vi "Imaging Data Display.vi"(0 "Frame number":i32, 9 "Filter gain":fxp<+,16,0>=0.8000030517578125, 11 "Kalman gain":fxp<+,16,1>=0.1015625) -> (4 "Image averaging done?":bool, 6 "Averaged image displayed?":bool, 8 "Frame imaging data Averaged?":bool, 10 "Averaged data address":u32, 14 "loop count":i32, 15 "Display_frames done":i32)   [LabVIEW 2015]
uses:
  <vilib>/Platform/TimedLoop/XDataNode/timing_clust.ctl
  <vilib>/Platform/TimedLoop/XDataNode/nitl_modes.ctl
  <vilib>/Platform/TimedLoop/XDataNode/wakeup.ctl
  <vilib>/rvi/Emulation/niFpgaGetClockAttributes.vi
  <vilib>/rvi/Emulation/niFpgaSctlEmulationGetInTimedLoop.vi
  <vilib>/rvi/Emulation/niFpgaEmulationReportErrorSimple.vi
  Globals/Global_Sample per Frame.vi
  <vilib>/rvi/Emulation/niFpgaCriticalErrorInLSC.vi
  <vilib>/rvi/DataTransferAndStorage/Container/Common/niFpgaContainerGetUniqueNameForEmu.vi
  <vilib>/rvi/DataTransferAndStorage/Container/Common/niFpgaContainerSetEmuInfo.vi
  <vilib>/rvi/eio/common/nirviEmuReportErrorAndStop.vi
  <vilib>/rvi/DataTransferAndStorage/Container/Common/niFpgaContainerExecOnDevCompGetState.vi
  <vilib>/rvi/Emulation/niFpgaEmulationIsFPGAContextNoSignature.vi
  <vilib>/rvi/errors/niFpgaSetErrorForExecOnDevCompSimple.vi
  <vilib>/rvi/FIFO/Fifo_Resource/nirvififoEmulationSetSize.vi
  <vilib>/rvi/FIFO/Fifo_Resource/nirviFifoEmulationQueueMgr.vi
  <instcachedir>/0/nirviFifoEmulationQueueMgr_E5CAEC123FF24DC58D834DCA3CDAA9B5.lvgen/nirviFifoEmulationQueueMgr_E5CAEC123FF24DC58D834DCA3CDAA9B5_002.vi
  <vilib>/rvi/FIFO/Fifo_Resource/nirvififoEmulationDetermineInputValidOut.vi
  <vilib>/rvi/FIFO/Fifo_Resource/nirvififoEmulationCreateLock.vi
  <vilib>/rvi/Emulation/niFpgaProcessEmulError.vi
  <vilib>/rvi/FIFO/Fifo_Resource/nirvififoEmulationObtainLock.vi
  <vilib>/rvi/FIFO/Fifo_Resource/nirvififoEmulationReleaseLock.vi
  <vilib>/rvi/occurrence/nirviWaitOnOccurrenceBase.vi
  <vilib>/rvi/errors/nirviReportUnexpectedCaseInternalError.vi
  <vilib>/rvi/errors/nirviReportUnexpectedCaseInternalError (U32).vi
  <vilib>/Utility/error.llb/Clear Errors.vi
  <vilib>/rvi/interface/RandomDataEmulation/niFpgaRandomDataHandleErrors.vi
  <vilib>/rvi/LocalResourceManager/LocalResourceManager.xnode
  <vilib>/rvi/DataTransferAndStorage/Container/XNode/niFpgaContainer.xnode
  <vilib>/rvi/FIFO/Fifo_Resource/niFpgaFifoEmulationRefIn.vi
  <vilib>/Platform/TimedLoop/XDataNode/XDataNode.xnode
  <vilib>/rvi/FIFO/Fifo_Resource/nirvififoEmulationWrite.vi
  <vilib>/rvi/FIFO/Fifo_Resource/nirvififoEmulationRead.vi
  <vilib>/Platform/TimedLoop/XDataNode/XDNodeRunTimeDep.lvlib
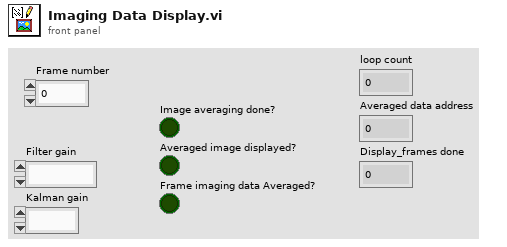
[diagram p1: front panel]
types:
  T1 = typedef "XDNodeRunTimeDep.lvlib/timing_clust.ctl" = cluster{"Expected End [f-1]":u64, "Actual End [f-1]":u64, "Finished Late? [f-1]":bool, "Expected End [i-1]":u64, "Actual End [i-1]":u64, "Finished Late? [i-1]":bool, "Expected Start [i]":u64, "Actual Start [i]":u64, "Expected Start [f]":u64, "Actual Start [f]":u64, "Source Name":string, "Structure Name":string, "Period":i64, "Deadline":i64, "Offset":i64, "Start":i64, "Priority":i32, "Timeout":i32, "Mode":T2, "Wakeup Reason":T3, "Error":errorcluster, "Source Type":string, "Secondary Source Type":string, "Global End Time":u64, "Global Start Time":u64, "Frame Duration":u64, "Iteration Duration":u64, "Assigned CPU":i32, "I/O Scan Engine Mode":u32}
  T2 = typedef "XDNodeRunTimeDep.lvlib/nitl_modes.ctl" = enum32{"No Change", "Process missed periods, maintain original phase", "Discard missed periods, maintain original phase", "Process missed periods, ignore original phase", "Discard missed periods, ignore original phase"}
  T3 = typedef "XDNodeRunTimeDep.lvlib/wakeup.ctl" = enum32{"Normal", "Aborted", "Asynchronous wakeup", "Timing source error", "Timed loop error", "Timeout"}
  T4 = cluster{"Numeric 1":u32, "Numeric 2":u32, "Numeric 3":u32, "Numeric 4":u32, "Numeric 5":u32, "Numeric 6":u32, "Numeric 7":u32, "Numeric 8":u32, "Numeric 9":u32, "Numeric 10":u32, "Numeric 11":u32, "Numeric 12":u32, "Numeric 13":u32, "Numeric 14":u32, "Numeric 15":u32, "Numeric 16":u32}
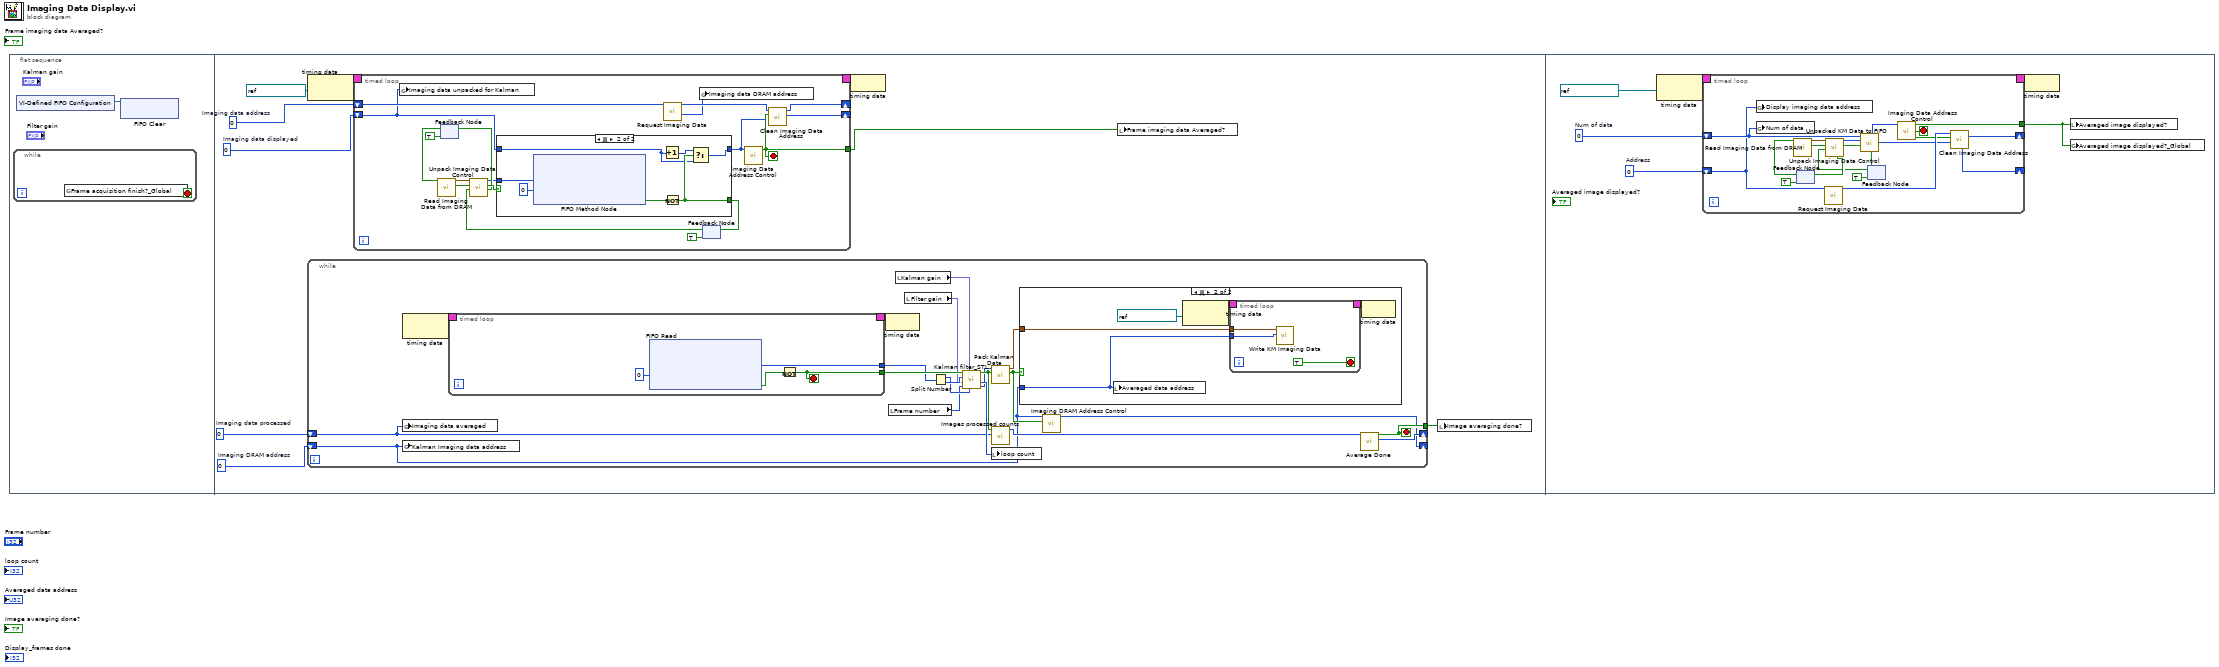
[diagram p0: block diagram]
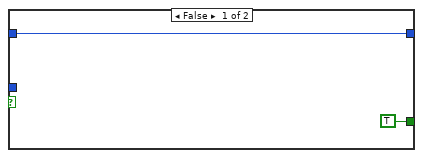
[diagram p3: hidden frame]
diagram:
  n1 = flat-sequence {
    frame #0 {
      n2 = while {
        stop <- w2 stop-if-true
        n3 = global read "Global_Sample per Frame.vi" "Frame acquisition finish?_Global"() -> (w2:bool)
      }
      n4 = xnode "VI-Defined FIFO Configuration"() -> ("FIFO输出"=w1:refnum<k21>)
      n5 = xnode ("FIFO Clear")("FIFO输入"=w1) -> ()  [unwired: 1 out]
    }
    frame #1 {
      w3 = u32 0  # Imaging DRAM address
      w6 = u32 0  # Imaging data processed
      w8 = u32 0  # Imaging data displayed
      w9 = u32 0  # Imaging data address
      n6 = node-c288(refnum<k21> "DRAM Clock" ("Source Name")) -> (w11:T1)
      n7 = while {
        shift-right: [w29] -> _
        shift-left: w6 -> [w15]
        tunnel: [w30] -> w4
        shift-right: [w17] -> _
        shift-left: w3 -> [w16]
        stop <- w30 stop-if-true
        n8 = node-c288() -> (w14:T1)  [unwired: 1 in]
        n9 = global write "Global_Sample per Frame.vi" "Imaging data averaged"(w15) -> ()
        n10 = global write "Global_Sample per Frame.vi" "Kalman Imaging data address"(w16) -> ()
        n11 = timed-loop {
          tunnel: [w32] -> w31
          tunnel: [w33] -> w27
          timing: w14 -> [_]
          timing-out: [_] -> w13
          stop <- w32 stop-if-true
          n12 = xnode ("FIFO Read")("超时"=0 ("Timeout")) -> ("元素"=w33:u32, "超时？"=w34:bool)  [unwired: 1 in, 1 out]
          n13 = Not(x=w34) -> (.not. x?=w32:bool)
        }
        n14 = node-c288(w13) -> ()
        n15 = local read "Frame number"() -> (w21:i32)
        n16 = local read "Kalman gain"() -> (w24:fxp<+,16,1>)
        n17 = local read "Filter gain"() -> (w23:fxp<+,16,0>)
        n18 = Split Number(x=w27) -> (hi(x)=w25:u16, lo(x)=w26:u16)
        n19 = call "Kalman filter_STL.vi"("Previous predicted pixel value"=w25, "Kalman gain"=w24, "Frame number"=w21, "Filter gain"=w23, "Pixel value"=w26, "Input valid"=w31) -> ("Kalman filter result"=w12:u16, "loop count"=w22:i32, "output valid"=w20:bool)  [unwired: 3 in]
        n20 = call "Pack Kalman Data.vi"("output valid"=w20, "Data"=w12) -> ("output valid?"=w18:bool, "packer out"=w19:T4)  [unwired: 8 in]
        n21 = call "Images processed counts.vi"("Imaging data processed in"=w15, "output valid"=w20) -> ("Imaging data processed out"=w28:u32)  [unwired: 9 in]
        n22 = local write "loop count"(w22) -> ()
        n23 = case shown="真" w18 {
          tunnel: w16 -> [_ w41]
          tunnel: w19 -> [_ w40]
          frame False {
          }
          frame True {
            n24 = local write "Averaged data address"(w41) -> ()
            n25 = node-c288(refnum<k21> "DRAM Clock" ("Source Name")) -> (w44:T1)
            n26 = timed-loop {
              timing: w44 -> [_]
              timing-out: [_] -> w43
              tunnel: w41 -> [w47]
              tunnel: w40 -> [w45]
              stop <- TRUE stop-if-true
              n27 = call "Write KM Imaging Data.vi"("Imaging DRAM address"=w47, "packer out"=w45) -> ()  [unwired: 10 in]
            }
            n28 = node-c288(w43) -> ()
          }
        }
        n29 = call "Imaging DRAM Address Control.vi"("output valid?"=w18, "Imaging DRAM address in"=w16) -> ("Imaging DRAM address out"=w17:u32)  [unwired: 9 in]
        n30 = call "Average Done.vi"("Imaging data processed"=w28) -> ("Imaging data address"=w29:u32, "Average Done"=w30:bool)  [unwired: 9 in]
      }
      n31 = timed-loop {
        shift-right: [w66] -> _
        shift-left: w9 -> [w56]
        timing: w11 -> [_]
        timing-out: [_] -> w10
        shift-right: [w65] -> _
        shift-left: w8 -> [w55]
        tunnel: [w69] -> w5
        stop <- w69 stop-if-true
        n32 = global write "Global_Sample per Frame.vi" "Imaging data unpacked for Kalman"(w55) -> ()
        n33 = feedback #1(TRUE) -> (w60:bool)
        n34 = call "Read Imaging Data from DRAM.vi"("Output ready"=w60) -> ("Output valid"=w59:bool, "Data"=w64:T4)  [unwired: 9 in]
        n35 = call "Request Imaging Data.vi"("Imaging data address in"=w56) -> ("Imaging data address in indicator"=w54:u32, "Imaging data address out"=w68:u32)  [unwired: 9 in]
        n36 = global write "Global_Sample per Frame.vi" "Imaging data DRAM address"(w54) -> ()
        n37 = feedback #2(TRUE) -> (w58:bool)
        n38 = call "Unpack Imaging Data Control.vi"("Output ready"=w58, "input valid"=w59, "Data"=w64) -> ("Input ready"=w62:bool, "output valid?"=w63:bool, "Unpacked data"=w57:u32)  [unwired: 6 in]
        n39 = feedback-in #1(w62) -> ()
        n40 = case shown="真" w63 {
          tunnel: [TRUE w77] -> w71
          tunnel: w57 -> [_ w74]
          tunnel: w55 -> [w72 w76]
          tunnel: [w72 w75] -> w67
          frame False {
          }
          frame True {
            n41 = xnode ("FIFO Method Node")("元素"=w74, "超时"=0 ("Timeout")) -> ("超时？"=w79:bool)  [unwired: 1 in, 1 out]
            n42 = Increment(x=w76) -> (x+1=w78:u32)
            n43 = Not(x=w79) -> (.not. x?=w77:bool)
            n44 = Select(t=w78, s=w77, f=w76) -> (s? t:f=w75:u32)
          }
        }
        n45 = feedback-in #2(w71) -> ()
        n46 = call "Imaging Data Address Control.vi"("Imaging data displayed"=w67) -> ("Clean"=w69:bool)  [unwired: 10 in]
        n47 = call "Clean Imaging Data Address.vi"("Imaging data displayed in"=w67, "Clean"=w69, "Imaging data address out"=w68) -> ("Imaging data displayed in"=w65:u32, "Imaging data address"=w66:u32)  [unwired: 7 in]
      }
      n48 = node-c288(w10) -> ()
      n49 = local write "Frame imaging data Averaged?"(w5) -> ()
      n50 = local write "Image averaging done?"(w4) -> ()
    }
    frame #2 {
      w89 = u32 0  # Address
      w90 = u32 0  # Num of data
      n51 = node-c288(refnum<k21> "DRAM Clock" ("Source Name")) -> (w92:T1)
      n52 = timed-loop {
        shift-right: [w96] -> _
        shift-left: w89 -> [w98]
        timing: w92 -> [_]
        timing-out: [_] -> w91
        shift-right: [w95] -> _
        shift-left: w90 -> [w107]
        tunnel: [w93] -> w87
        stop <- w93 stop-if-true
        n53 = global write "Global_Sample per Frame.vi" "Display imaging data address"(w98) -> ()
        n54 = global write "Global_Sample per Frame.vi" "Num of data"(w107) -> ()
        n55 = feedback #3(TRUE) -> (w102:bool)
        n56 = call "Read Imaging Data from DRAM.vi"("Output ready"=w102) -> ("Output valid"=w105:bool, "Data"=w106:T4)  [unwired: 9 in]
        n57 = call "Request Imaging Data.vi"("Imaging data address in"=w98) -> ("Imaging data address out"=w97:u32)  [unwired: 9 in, 1 out]
        n58 = feedback #4(TRUE) -> (w101:bool)
        n59 = call "Unpack Imaging Data Control.vi"("Output ready"=w101, "input valid"=w105, "Data"=w106) -> ("Input ready"=w103:bool, "output valid?"=w100:bool, "Unpacked data"=w99:u32)  [unwired: 6 in]
        n60 = feedback-in #3(w103) -> ()
        n61 = call "Unpacked KM Data to FIFO.vi"("output valid?"=w100, "Unpacked data"=w99, "Num of data in"=w107) -> ("in time"=w109:bool, "Num of data out"=w94:u32)  [unwired: 7 in]
        n62 = feedback-in #4(w109) -> ()
        n63 = call "Imaging Data Address Control.vi"("Imaging data displayed"=w94) -> ("Clean"=w93:bool)  [unwired: 10 in]
        n64 = call "Clean Imaging Data Address.vi"("Imaging data displayed in"=w94, "Clean"=w93, "Imaging data address out"=w97) -> ("Imaging data displayed in"=w95:u32, "Imaging data address"=w96:u32)  [unwired: 7 in]
      }
      n65 = node-c288(w91) -> ()
      n66 = local write "Averaged image displayed?"(w87) -> ()
      n67 = global write "Global_Sample per Frame.vi" "Averaged image displayed?_Global"(w87) -> ()
    }
  }
